vi "Launcher GUI Setting.vi"(8 "error in (no error)":errorcluster, 11 "VI in":refnum<vi>) -> (0 "error out":errorcluster, 3 "VI out":refnum<vi>)   [LabVIEW 2018]
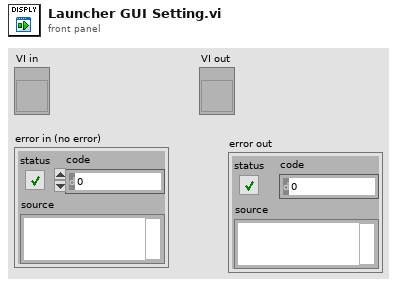
[diagram p1: front panel]
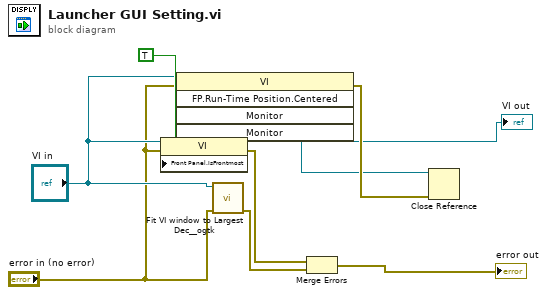
[diagram p0: block diagram]
diagram:
  n1 = property class="VI"(reference="VI in", error in="error in (no error)", "Front Panel.IsFrontmost"=TRUE ("Front Panel Window:Is Frontmost")) -> (reference out=→"VI out":refnum<vi>, error out=w8:errorcluster)
  n2 = invoke class="VI" method="FP.Run-Time Position.Centered"(reference="VI in", error in="error in (no error)") -> (reference out=w6:refnum<vi>, error out=w9:errorcluster)  [unwired: 3 in, 3 out]
  n3 = call <userlib>:"Fit VI window to Largest Dec__ogtk.vi"("error in (no error)"="error in (no error)", "VI Ref (calling VI)"="VI in") -> ("error out"=w2:errorcluster)  [unwired: 4 in, 1 out]
  n4 = Merge Errors(w8, w2) -> (→"error out":errorcluster)
  n5 = Close Reference(reference=w6, error in (no error)=w9) -> ()  [unwired: 1 out]
